vi "TDC_getDeviceParams.vi"(8 "Error In":errorcluster) -> (0 "Error Out":errorcluster, 1 "Exposure Time [ms]":i32, 2 "Coincidence Window [bins]":i32, 3 "Channel Mask":i32)   [LabVIEW 2011]
uses:
  dist/userlib/lib/tdcbase.dll
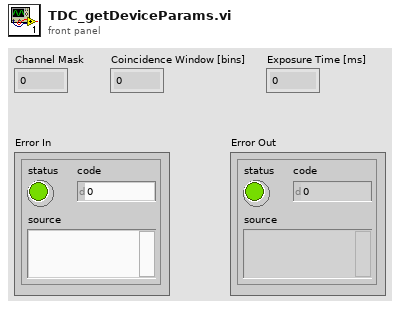
[diagram p1: front panel]
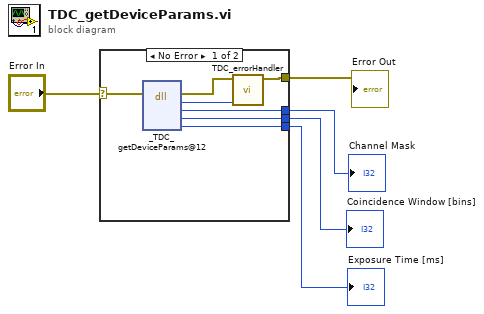
[diagram p0: block diagram]
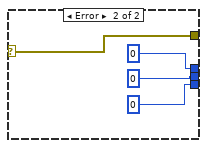
[diagram p2: hidden frame]
diagram:
  n1 = case shown="No Error" "Error In" {
    selector: "Error In" -> [w9 w16]
    tunnel: [w6 w16] -> w4
    tunnel: [w12 0] -> w3
    tunnel: [w11 0] -> w2
    tunnel: [w10 0] -> w1
    frame No Error {
      n2 = dll-call lib="C:/nh/projekt/spmctrl/dist/userlib/lib/tdcbase.dll" fn="_TDC_getDeviceParams@12"(error in=w9) -> (error out=w8:errorcluster, "return type"=w7:i32, "channelMask"=w12:i32, "coincWin"=w11:i32, "expTime"=w10:i32)  [unwired: 5 in, 1 out]
      n3 = call "TDC_errorHandler.vi"("quTAU Return Code"=w7, "Error In"=w8) -> ("Error Out"=w6:errorcluster)  [unwired: 9 in]
    }
    frame Error {
    }
  }
  "Error Out" <- w4
  "Channel Mask" <- w3
  "Coincidence Window [bins]" <- w2
  "Exposure Time [ms]" <- w1
